vi "DriveWaitForManip.vi"(2 "Parameter String":string) -> (0 "Error Out":errorcluster, 1 "Increment":bool)   [LabVIEW 2020]
doc: "This VI pauses the drive sequencer until the manipulator sequencer has reached (or passed) the specified step.\n\nParameters:\nParam1: manipulator step to wait for"
uses:
  SafeParser_Integer.vi
  drivercommands.vi
  autonomousinfo.vi
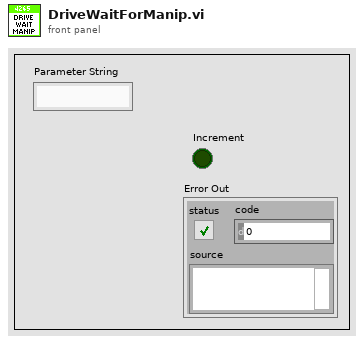
[diagram p1: front panel]
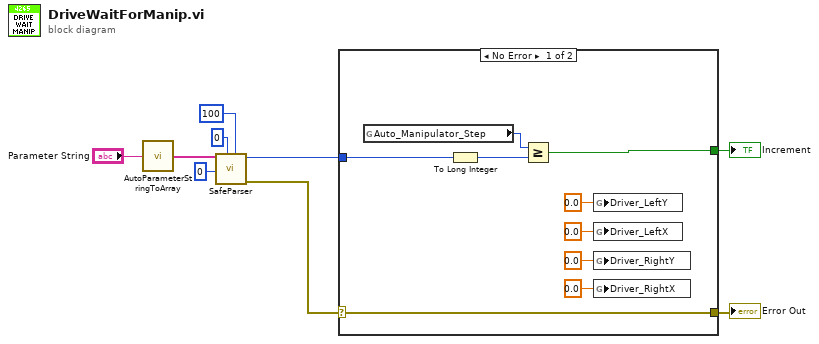
[diagram p0: block diagram]
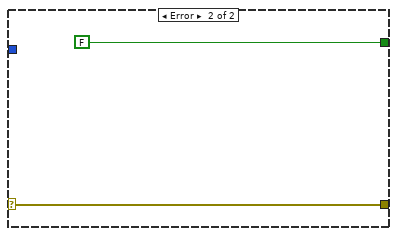
[diagram p2: hidden frame]
diagram:
  n1 = call "AutoParameterStringToArray.vi"("Parameter String"="Parameter String") -> ("Parsed Parameters"=w2:string[])
  n2 = call-poly "SafeParser.vi"("Maximum"=100, "Minimum"=0, "Array Index"=0 ("Parameter Index"), "String Array"=w2) -> ("Error Out"=w1:errorcluster, "Typecast  Value"=w6:i32)  [unwired: 6 in]
  n3 = case shown="No Error" w1 {
    selector: w1 -> [w14 w20]
    tunnel: [w10 FALSE] -> w9
    tunnel: [w14 w20] -> w8
    tunnel: w6 -> [w11 _]
    frame No Error {
      n4 = global read "autonomousinfo.vi" "Auto_Manipulator_Step"() -> (w13:i32)
      n5 = To Long Integer(number=w11) -> (32bit integer=w12:i32)
      n6 = Greater Or Equal?(x=w13, y=w12) -> (x >= y?=w10:bool)
      n7 = global write "drivercommands.vi" "Driver_LeftY"(0.0 ("Driver_LeftY")) -> ()
      n8 = global write "drivercommands.vi" "Driver_LeftX"(0.0 ("Driver_RightX")) -> ()
      n9 = global write "drivercommands.vi" "Driver_RightY"(0.0 ("Driver_RightX")) -> ()
      n10 = global write "drivercommands.vi" "Driver_RightX"(0.0 ("Driver_RightX")) -> ()
    }
    frame Error {
    }
  }
  "Increment" <- w9
  "Error Out" <- w8
